vi "SetFileFlowScript.vi"(8 "error in (no error)":errorcluster, 11 "Fileflow script":string[](array[string])) -> (0 "error out":errorcluster)   [LabVIEW 2017, in "FileFlow.lvlib"]
uses:
  <vilib>/addons/InsightCM/Devices/Shared/Common/FileFlow/FileFlow.lvlib
  <vilib>/addons/PointValueMap/subVIs/Point_Write_variant.vi
  <vilib>/addons/InsightCM/Utilities/GlobalConfiguration/GlobalConfiguration.lvlib
  <vilib>/addons/PointValueMap/PointValueMap.lvlib
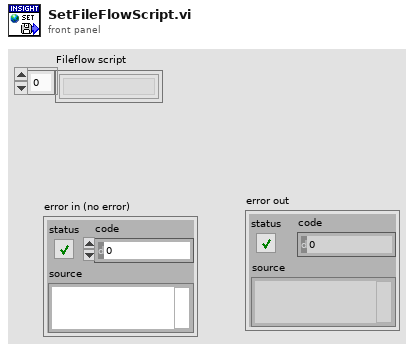
[diagram p1: front panel]
types:
  T1 = typedef "PointValueMap.lvlib/PointMap.ctl" = refnum<data-value>
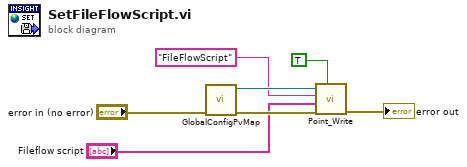
[diagram p0: block diagram]
diagram:
  n1 = call <vilib>:"GlobalConfigPvMap.vi"("error in (no error)"="error in (no error)") -> ("error out"=w6:errorcluster, "global configuration map"=w5:T1)  [unwired: 9 in]
  n2 = call-poly <vilib>:"Point_Write.vi"("Auto Create?"=TRUE, "Error In"=w6, "Value"="Fileflow script", "Tag"="FileFlowScript" ("Name"), "Map"=w5) -> ("Error Out"=→"error out":errorcluster)  [unwired: 5 in, 1 out]
